vi "Test Waveform Diogo_CD.vi"() -> ()   [LabVIEW 2016]
uses:
  <vilib>/xnet/xnet.llb/XNET Read (Signal Waveform) .vi
  <vilib>/measure/matone.llb/Extract Single Tone Information 1 Chan.vi
  <vilib>/Waveform/WDTOps.llb/WDT Append Waveforms DBL.vi
  <vilib>/Waveform/WDTOps.llb/WDT Number of Waveform Samples DBL.vi
  <vilib>/measure/NI_MAPro.lvlib
panel:
  in  "signal type":T1(ring)
  out "test passed?":bool
  out "error out 3":errorcluster
  out "error out 2":errorcluster caption="error out"
  out "error out":errorcluster
  out "Waveform Graph":waveform(dbl)[](graph)
  in  "stop":bool
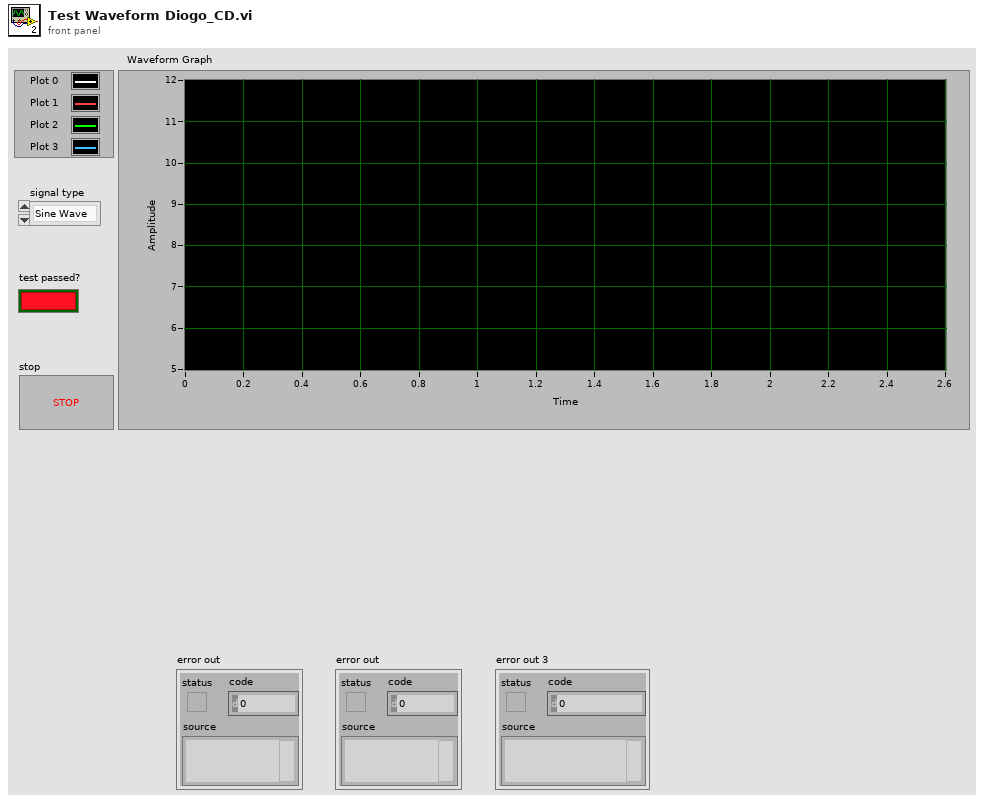
[diagram p1: front panel]
types:
  T1 = enum16{"Sine Wave", "Triangle Wave", "Square Wave", "Sawtooth Wave"}
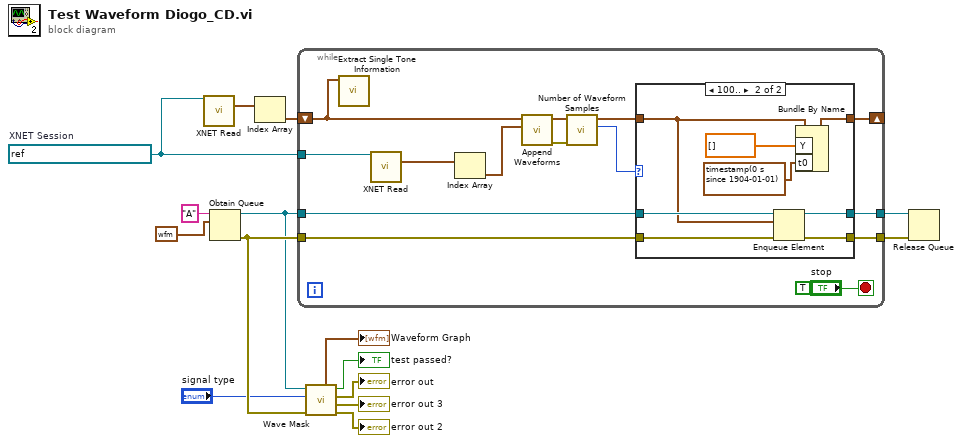
[diagram p0: block diagram]
diagram:
  w9 = refnum<k21> "New NI-XNET Session"  # XNET Session
  n1 = call-poly <vilib>:"XNET Read.vi"("session in"=w9) -> ("data"=w10:waveform(dbl)[])  [unwired: 12 in, 2 out]
  n2 = Obtain Queue(name (unnamed)="A", element data type=waveform(dbl) {"t0"=timestamp(0 s since 1904-01-01), "dt"=1.0, "Y"=[]}) -> (queue out=w11:refnum<queue>, error out=w12:errorcluster)  [unwired: 3 in, 1 out]
  n3 = Index Array(array=w10) -> (element=w8:waveform(dbl))  [unwired: 1 in]
  n4 = while {
    tunnel: w9 -> [w29]
    tunnel: w11 -> [w27]
    tunnel: [w26] -> w15
    tunnel: [w25] -> w7
    tunnel: w12 -> [w24]
    shift-right: [w17] -> _
    shift-left: w8 -> [w16]
    stop <- "stop" stop-if-true
    (unwired) TRUE
    n5 = call-poly <vilib>:"Extract Single Tone Information.vi"("time signal in"=w16) -> ()  [unwired: 5 in, 6 out]
    n6 = call-poly <vilib>:"XNET Read.vi"("session in"=w29) -> ("data"=w23:waveform(dbl)[])  [unwired: 12 in, 2 out]
    n7 = Index Array(array=w23) -> (element=w22:waveform(dbl))  [unwired: 1 in]
    n8 = call-poly <vilib>:"Append Waveforms.vi"("waveform B"=w22, "waveform A"=w16) -> ("error out"=w21:errorcluster, "waveform out"=w20:waveform(dbl))  [unwired: 8 in]
    n9 = call-poly <vilib>:"Number of Waveform Samples.vi"("error in (no error)"=w21, "waveform in"=w20) -> ("number of samples"=w19:i32, "waveform out"=w18:waveform(dbl))  [unwired: 7 in, 1 out]
    n10 = case shown="100.." w19 {
      tunnel: w27 -> [w31 w40]
      tunnel: [w31 w39] -> w26
      tunnel: [w30 w38] -> w25
      tunnel: w24 -> [w30 w37]
      tunnel: w18 -> [w32 w36]
      tunnel: [w32 w35] -> w17
      frame 0, Default {
      }
      frame 100.. {
        n11 = Enqueue Element(queue=w40, element=w36, error in (no error)=w37) -> (queue out=w39:refnum<queue>, error out=w38:errorcluster)  [unwired: 1 in, 1 out]
        n12 = Bundle By Name(cluster=w36, "Y"=dbl[] [], "t0"=timestamp(0 s since 1904-01-01)) -> (w35:waveform(dbl))
      }
    }
  }
  n13 = call "Wave Mask.vi"("error in (no error)"=w12, "signal type"="signal type", "Queue in"=w11) -> ("error out"=→"error out 2":errorcluster, "error out 3"=→"error out 3":errorcluster, "error out 2"=→"error out":errorcluster, "test passed?"=→"test passed?":bool, "output values"=→"Waveform Graph":waveform(dbl)[])  [unwired: 4 in]
  n14 = Release Queue(queue=w15, error in (no error)=w7) -> ()  [unwired: 1 in, 3 out]
